vi "Initialize.vi"(8 "error in":errorcluster, 9 "Path":path, 10 "Device":string, 11 "Config in":refnum<class "Config.lvclass">) -> (0 "error out":errorcluster, 3 "Config out":refnum<class "Config.lvclass">)   [LabVIEW 2023, in "Config.lvlib" / "Config.lvclass"]
doc: "The configuration Initiailize.vi is used to load default settings for any device (instrument, communications protocol, etc) and return default configurable values to the caller class.\n\nThis utility allows for on the fly hardware changes without requiring modification to the test software. It creates a nearly plug and play diversity to instrument and communication bus drivers, known as an abstraction layer. \n\nFurther, this utility can be built out as a packed project library (PPL) which prevents the end user from modifying the test code, preventing any risk of operator invalidation of the test. PPLs are also stored in a binary format and as a result require substantially less memory and load times at the initialization of a test."
uses:
  Config.lvclass
  Config.lvclass/Config.ctl
  Accessors/Write Path.vi
  Accessors/Read Path.vi
  Private/Write Signal List.vi
  Accessors/Write Device.vi
  builds/Tools/SLL.lvlibp/SLL.lvclass
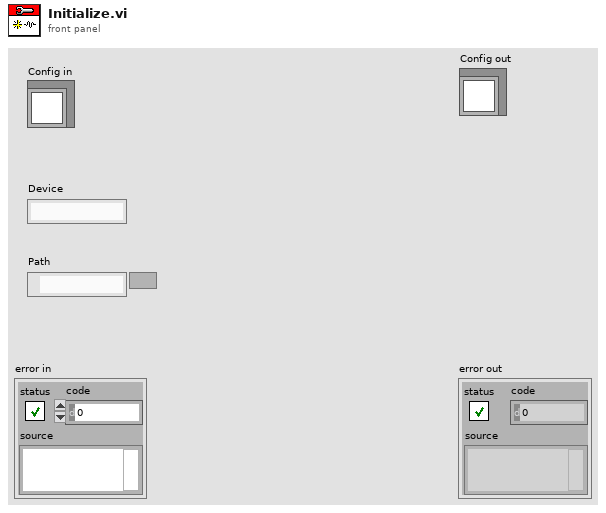
[diagram p1: front panel]
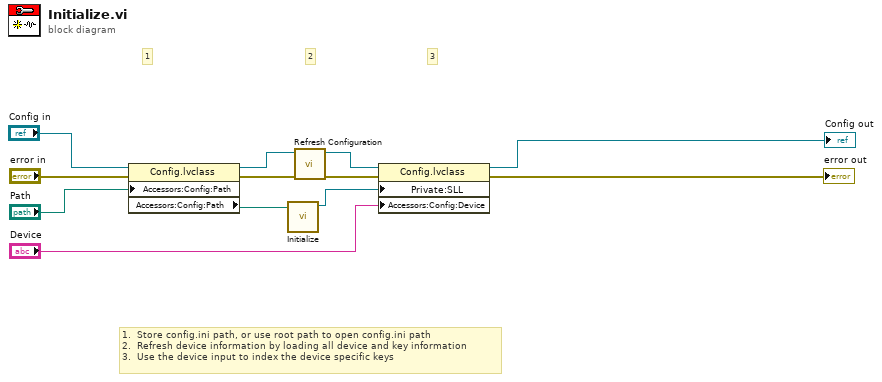
[diagram p0: block diagram]
diagram:
  # "1.  Store config.ini path, or use root path to open config.ini path\n2.  Refresh device information by loading all device and key information\n3.  Use the device input to index the device specific keys"
  # "3"
  # "2"
  # "1"
  n1 = property class="Config.lvclass"(reference="Config in", error in="error in", "Accessors:Config:Path"="Path") -> (reference out=w9:refnum<class "Config.lvclass">, error out=w8:errorcluster, "Accessors:Config:Path"=w3:path)
  n2 = call "Initialize.vi"("Application Directory"=w3) -> ("SLL out"=w1:refnum<class "SLL.lvclass">)  [unwired: 9 in, 1 out]
  n3 = call "Refresh Configuration.vi"("error in"=w8, "Config in"=w9) -> ("error out"=w6:errorcluster, "Config out"=w7:refnum<class "Config.lvclass">)  [unwired: 8 in]
  n4 = property class="Config.lvclass"(reference=w7, error in=w6, "Private:SLL"=w1, "Accessors:Config:Device"="Device") -> (reference out=→"Config out":refnum<class "Config.lvclass">, error out=→"error out":errorcluster)
